vi "pH Controller v1_0 July 2016.vi"() -> ()   [LabVIEW 2012]
uses:
  <vilib>/Utility/file.llb/Write To Spreadsheet File (DBL).vi
panel:
  out "array":dbl[](array[numeric])
  in  "Reset Time, Ti (s)":dbl(slide) min=0.0 max=120.0 step=0.001 scale=0.0..120.0 scale format="%_3g"
  in  "Controller Gain, Kc":dbl(slide) min=0.0 max=120.0 step=0.001 scale=0.0..120.0 scale format="%_3g"
  in  "Derivative Time, Td (s)":dbl(slide) min=0.0 max=120.0 step=0.001 scale=0.0..120.0 scale format="%_3g"
  in  "Time (s)":dbl=0.25 min=0.01 step=0.01 format="%.2g"
  out "Time (s)":dbl
  in  "Stop and Save":bool
  out "Pump indicator":bool
  out "Contoller Output %":dbl(slide) scale=-100.0..100.0
  in  "Set Value":dbl=7.0 min=0.0 max=14.0 step=0.01 format="%.2f"
  out "pH vs. Time":cluster{"Ave pH":dbl, "Set Value":dbl}(graph)
  # "UCSD CENG 176\npH Controller"
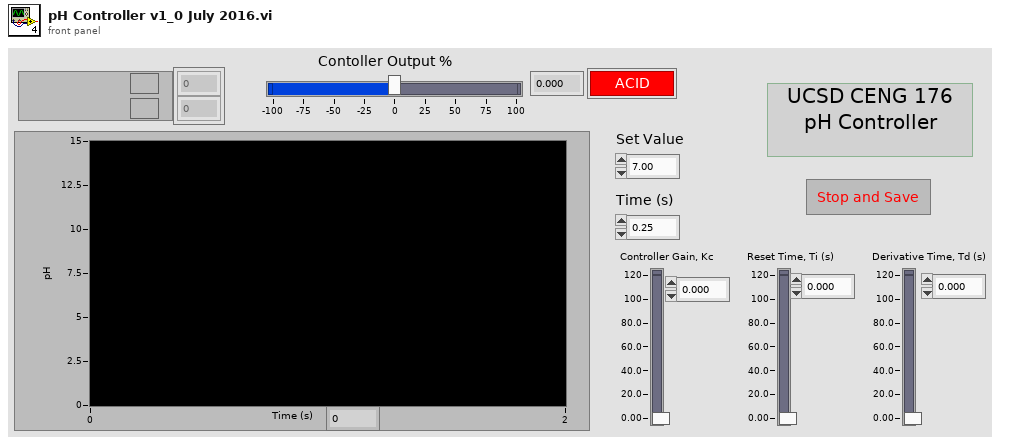
[diagram p1: front panel]
types:
  T1 = cluster{"Controller Gain, Kc":dbl, "Reset Time, Ti (s) ":dbl, "Derivative Time, Td (s)":dbl}
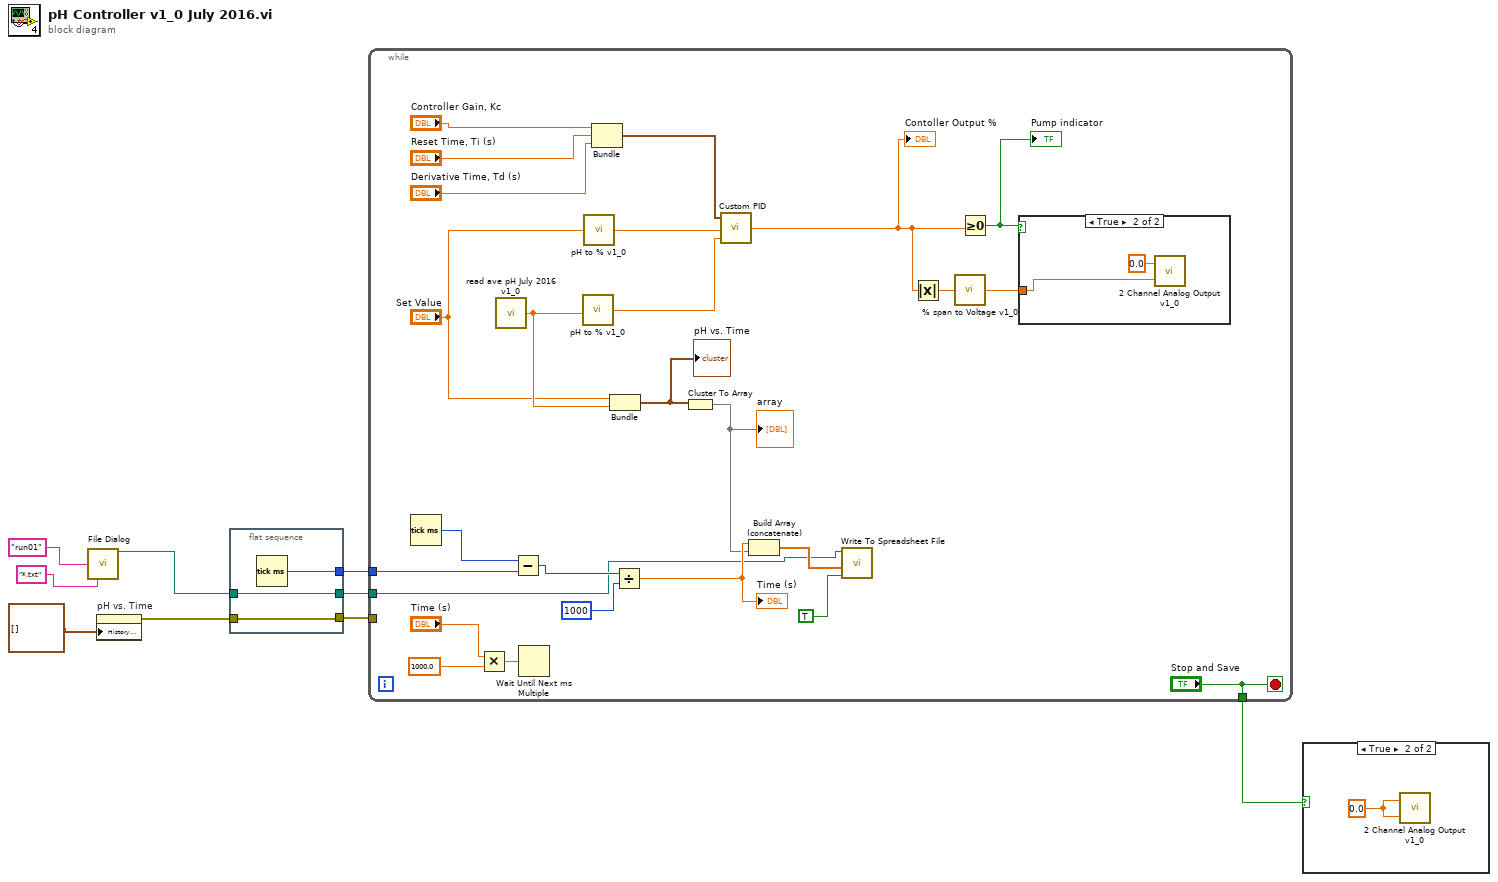
[diagram p0: block diagram]
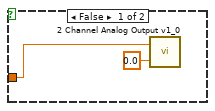
[diagram p3: hidden frame]
diagram:
  n1 = call "File Dialog"("default name"="run01", "pattern (all files)"="*.txt" ("pattern label")) -> ("selected path"=w7:path)  [unwired: 10 in, 3 out]
  n2 = property on="pH vs. Time" class="WFChart (strict)"("History Data"=cluster{"Ave pH":dbl, "Set Value":dbl}[] []) -> (error out=w4:errorcluster)  [unwired: 2 in, 1 out]
  n3 = flat-sequence {
    tunnel: w7 -> [w11]
    tunnel: [w12] -> w6
    tunnel: [w11] -> w5
    tunnel: w4 -> [w10]
    tunnel: [w10] -> w3
    frame #0 {
      n4 = Tick Count (ms)() -> (millisecond timer value=w12:u32)
    }
  }
  n5 = while {
    tunnel: ["Stop and Save"] -> w9
    tunnel: w6 -> [w31]
    tunnel: w5 -> [w20]
    tunnel: w3 -> [_]
    stop <- "Stop and Save" stop-if-true
    n6 = Tick Count (ms)() -> (millisecond timer value=w30:u32)
    n7 = Multiply(x="Time (s)", y=1000.0) -> (x*y=w23:dbl)
    n8 = call "read ave pH July 2016 v1_0.vi"() -> ("Ave pH"=w14:dbl)  [unwired: 1 in]
    n9 = Subtract(x=w30, y=w31) -> (x-y=w29:u32)
    n10 = Wait Until Next ms Multiple(millisecond multiple=w23) -> ()  [unwired: 1 out]
    n11 = call "pH to % v1_0.vi"("Input pH"=w14) -> ("Output Percentage"=w37:dbl)  [unwired: 2 in]
    n12 = call "pH to % v1_0.vi"("Input pH"="Set Value") -> ("Output Percentage"=w38:dbl)  [unwired: 2 in]
    n13 = Bundle("Controller Gain, Kc"="Controller Gain, Kc", "Reset Time, Ti (s)"="Reset Time, Ti (s)", "Derivative Time, Td (s)"="Derivative Time, Td (s)") -> (w16:T1)  [unwired: 1 in]
    n14 = Bundle("Set Value"="Set Value", "Ave pH"=w14) -> (w15:cluster{"Set Value":dbl, "Ave pH":dbl})  [unwired: 1 in]
    "pH vs. Time" <- w15
    n15 = Divide(x=w29, y=1000) -> (x/y=w26:dbl)
    "Time (s)" <- w26
    n16 = Cluster To Array(cluster=w15) -> (array=w25:dbl[])
    "array" <- w25
    n17 = call "Custom PID.vi"("Present Value"=w37, "Set Point"=w38, "Tuning Parameters"=w16) -> ("Controller Output"=w34:dbl)
    "Contoller Output %" <- w34
    n18 = Build Array (concatenate)(w26, w25) -> (w24:dbl[])
    n19 = call-poly <vilib>:"Write To Spreadsheet File.vi"("append to file? (new file:F)"=TRUE, "1D data"=w24, "file path (dialog if empty)"=w20) -> ()  [unwired: 5 in, 1 out]
    n20 = Absolute Value(x=w34) -> (abs(x)=w35:dbl)
    n21 = call "% span to Voltage v1_0.vi"("% span"=w35) -> ("Output Voltage"=w33:dbl)  [unwired: 2 in]
    n22 = Greater Or Equal To 0?(x=w34) -> (x >= 0?=w36:bool)
    "Pump indicator" <- w36
    n23 = case shown="True" w36 {
      tunnel: w33 -> [w39 w41]
      frame False {
        n24 = call "2 Channel Analog Output v1_0.vi"("Voltage output 1"=0.0, "Voltage output 0"=w39) -> ()  [unwired: 1 in]
      }
      frame True {
        n25 = call "2 Channel Analog Output v1_0.vi"("Voltage output 1"=w41, "Voltage output 0"=0.0) -> ()  [unwired: 1 in]
      }
    }
  }
  n26 = case shown="True" w9 {
    frame False {
    }
    frame True {
      w43 = 0.0 ("Voltage output 1")
      n27 = call "2 Channel Analog Output v1_0.vi"("Voltage output 1"=w43, "Voltage output 0"=w43) -> ()  [unwired: 1 in]
    }
  }
